vi "Send Loop Metrics.vi"(8 "error in (no error)":errorcluster, 11 "Module in":refnum<class "Module.lvclass">) -> (0 "error out":errorcluster, 3 "Module out":refnum<class "Module.lvclass">)   [LabVIEW 2020, in "Volatus.lvlib" / "Module.lvclass"]
uses:
  Module.lvclass
  Module.lvclass/Module.ctl
  MessageQ/MessageQ.lvclass/MessageQ.ctl
  Forward Metric.vi
  Parent Q.vi
  MessageQ/Is Null.vi
  MessageQ/Send.vi
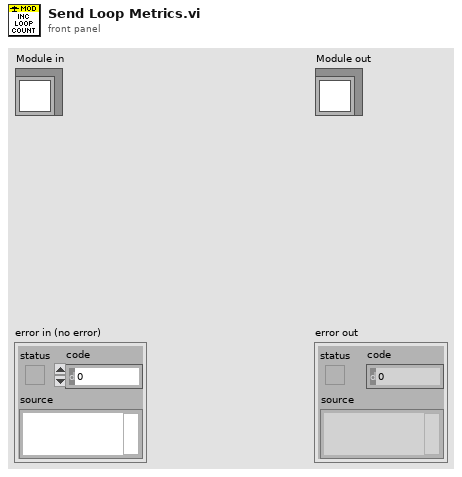
[diagram p1: front panel]
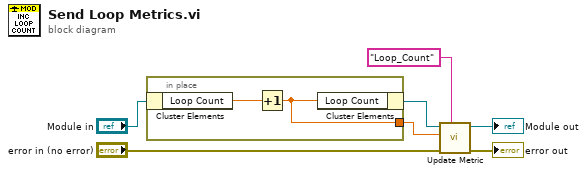
[diagram p0: block diagram]
diagram:
  n1 = in-place {
    in-place-border: [w8] -> w1
    n2 = in-place-cluster #1("Module in") -> ("Loop Count"=w9:dbl)
    n3 = Increment(x=w9) -> (x+1=w8:dbl)
    n4 = in-place-cluster #1("Loop Count"=w8) -> (w4:refnum<class "Module.lvclass">)
  }
  n5 = call "Update Metric.vi"("Metric"="Loop_Count", "error in (no error)"="error in (no error)", "Value"=w1, "Module in"=w4) -> ("error out"=→"error out":errorcluster, "Module out"=→"Module out":refnum<class "Module.lvclass">)  [unwired: 6 in]
